vi "Configure Trigger (Runt).vi"(0 "VISA resource name":refnum<visa-resource-name>, 1 "Polarity (0:Positive)":u16(ring) items=["Positive", "Negative", "Either"], 2 "Upper Level (1.2V)":dbl=1.2, 3 "Lower Level (0.8V)":dbl=0.8, 5 "Source (0:Channel1)":u16(ring) items=["Channel1", "Channel2", "Channel3", "Channel4", "Digital Channel0", "Digital Channel1", "Digital Channel2", "Digital Channel3", "Digital Channel4", "Digital Channel5", "Digital Channel6", "Digital Channel7", "Digital Channel8", "Digital Channel9", "Digital Channel10", "Digital Channel11", "Digital Channel12", "Digital Channel13", "Digital Channel14", "Digital Channel15"], 7 "Trigger Condition (1: Wider than)":u16(ring)=1 items=["Occurs", "Wider Than"], 9 "Runt Width (500E-12s)":dbl=5e-10, 11 "error in (no error)":errorcluster, 12 "Trigger if Runt (0:Occurs)":u16(ring) items=["Occurs", "Logic", "Bus"], 13 "Trigger Event (0:A Event)":u16(ring) items=["A Event", "B Event"]) -> (4 "VISA resource name out":refnum<visa-resource-name>, 6 "Trigger Event Out":u16(ring) items=["A Event", "B Event"], 15 "error out":errorcluster)   [LabVIEW 2012, in "Tektronix 7000 Series.lvlib"]
doc: "Configures Runt trigger settings for an oscilloscope.A runt occurs when the oscilloscope detects a positive or negative going pulse that crosses one voltage threshold but fails to cross a second threshold before re-crossing the first. \n\nTDS5000,TDS5000B,TDS6000,CSA7000 and TDS7000 series oscilloscopes don't support B Runt Trigger."
uses:
  Tektronix 7000 Series.lvlib
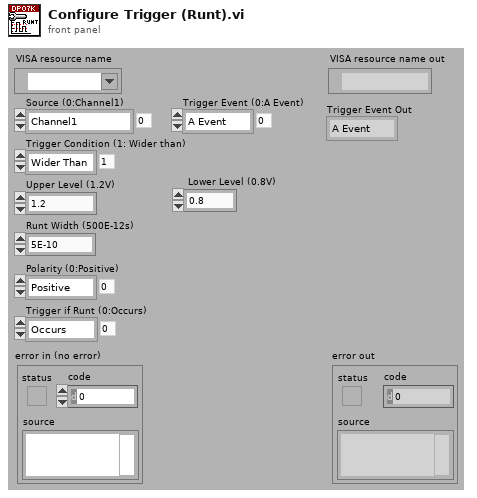
[diagram p1: front panel]
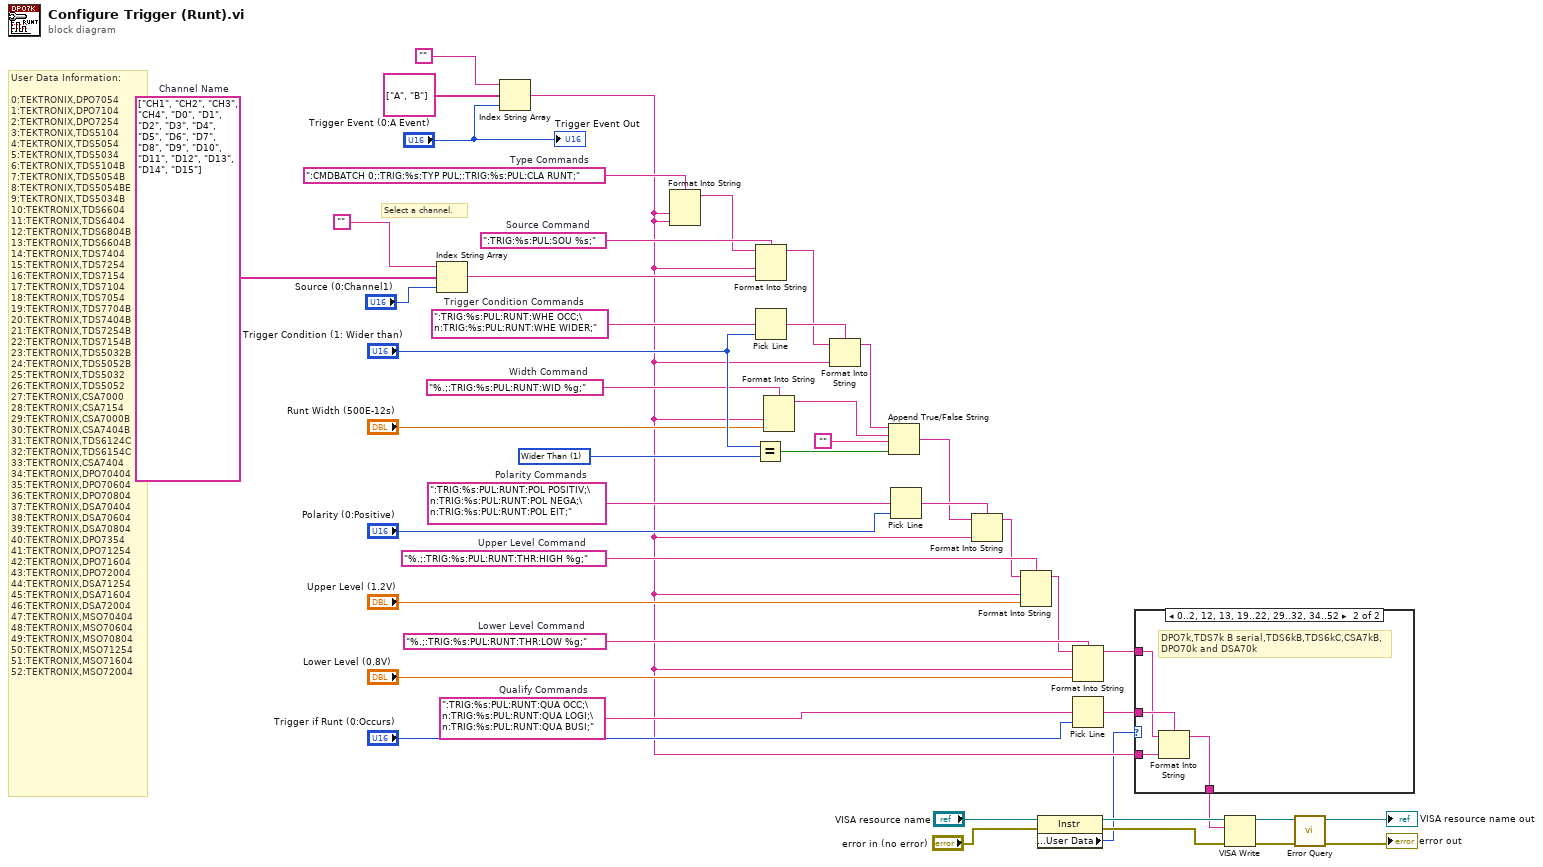
[diagram p0: block diagram]
diagram:
  w1 = string[] ["CH1", "CH2", "CH3", "CH4", "D0", "D1", "D2", "D3", "D4", "D5", "D6", "D7", "D8", "D9", "D10", "D11", "D12", "D13", "D14", "D15"]  # Channel Name
  w27 = "%.;:TRIG:%s:PUL:RUNT:WID %g;"  # Width Command
  w28 = u16 1 items=["Occurs", "Wider Than"] ("Trigger Condition (1: Wider than)")
  w30 = ":TRIG:%s:PUL:RUNT:QUA OCC;\n:TRIG:%s:PUL:RUNT:QUA LOGI;\n:TRIG:%s:PUL:RUNT:QUA BUSI;"  # Qualify Commands
  w31 = ":TRIG:%s:PUL:RUNT:POL POSITIV;\n:TRIG:%s:PUL:RUNT:POL NEGA;\n:TRIG:%s:PUL:RUNT:POL EIT;"  # Polarity Commands
  w33 = ":TRIG:%s:PUL:RUNT:WHE OCC;\n:TRIG:%s:PUL:RUNT:WHE WIDER;"  # Trigger Condition Commands
  w32 = "%.;:TRIG:%s:PUL:RUNT:THR:LOW %g;"  # Lower Level Command
  w34 = "%.;:TRIG:%s:PUL:RUNT:THR:HIGH %g;"  # Upper Level Command
  w35 = ":TRIG:%s:PUL:SOU %s;"  # Source Command
  w23 = ":CMDBATCH 0;:TRIG:%s:TYP PUL;:TRIG:%s:PUL:CLA RUNT;"  # Type Commands
  # "User Data Information:\n\n0:TEKTRONIX,DPO7054\n1:TEKTRONIX,DPO7104\n2:TEKTRONIX,DPO7254\n3:TEKTRONIX,TDS5104\n4:TEKTRONIX,TDS5054\n5:TEKTRONIX,TDS5034\n6:TEKTRONIX,TDS5104B\n7:TEKTRONIX,TDS5054B\n8:TEKTRONIX,TDS5054BE\n9:TEKTRONIX,TDS5034B\n10:TEKTRONIX,TDS6604\n11:TEKTRONIX,TDS6404\n12:TEKTRONIX,TDS6804B\n13:TEKTRONIX,TDS6604B\n14:TEKTRONIX,TDS7404\n15:TEKTRONIX,TDS7254\n16:TEKTRONIX,TDS7154\n17:TEKTRONIX,TDS7104\n18:TEKTRONIX,TDS7054\n19:TEKTRONIX,TDS7704B\n20:TEKTRONIX,TDS7404B\n21:TEKTRONIX,TDS7254B\n22:TEKTRONIX,TDS7154B\n23:TEKTRONIX,TDS5032B\n24:TEKTRONIX,TDS5052B\n25:TEKTRONIX,TDS5032\n26:TEKTRONIX,TDS5052\n27:TEKTRONIX,CSA7000\n28:TEKTRONIX,CSA7154\n29:TEKTRONIX,CSA7000B\n30:TEKTRONIX,CSA7404B\n31:TEKTRONIX,TDS6124C\n32:TEKTRONIX,TDS6154C\n33:TEKTRONIX,CSA7404\n34:TEKTRONIX,DPO70404\n35:TEKTRONIX,DPO70604\n36:TEKTRONIX,DPO70804\n37:TEKTRONIX,DSA70404\n38:TEKTRONIX,DSA70604\n39:TEKTRONIX,DSA70804\n40:TEKTRONIX,DPO7354\n41:TEKTRONIX,DPO71254\n42:TEKTRONIX,DPO71604\n43:TEKTRONIX,DPO72004\n44:TEKTRONIX,DSA71254\n45:TEKTRONIX,DSA71604\n46:TEKTRONIX,DSA72004\n47:TEKTRONIX,MSO70404\n48:TEKTRONIX,MSO70604\n49:TEKTRONIX,MSO70804\n50:TEKTRONIX,MSO71254\n51:TEKTRONIX,MSO71604\n52:TEKTRONIX,MSO72004"
  # "Select a channel."
  n1 = Index String Array(1:"Source (0:Channel1)", 2:w1, 3:"" ("Empty String Constant")) -> (0:w22:string)
  n2 = Index String Array(1:"Trigger Event (0:A Event)", 2:string[] ["A", "B"], 3:"" ("Empty String Constant")) -> (0:w6:string)
  n3 = Format Into String(format string=w23, w6, w6) -> (resulting string=w21:string)  [unwired: 2 in, 1 out]
  n4 = Equal?(x="Trigger Condition (1: Wider than)", y=w28) -> (x = y?=w26:bool)
  n5 = Format Into String(format string=w35, initial string=w21, w6, w22) -> (resulting string=w19:string)  [unwired: 1 in, 1 out]
  n6 = Pick Line(multi-line string=w33, line index="Trigger Condition (1: Wider than)") -> (output string=w20:string)  [unwired: 1 in]
  n7 = Format Into String(format string=w27, w6, "Runt Width (500E-12s)") -> (resulting string=w25:string)  [unwired: 2 in, 1 out]
  n8 = Format Into String(format string=w20, initial string=w19, w6) -> (resulting string=w17:string)  [unwired: 1 in, 1 out]
  n9 = Append True/False String(1:w26, 2:"" ("Empty String Constant"), 3:w25, 4:w17) -> (0:w15:string)
  n10 = Pick Line(multi-line string=w31, line index="Polarity (0:Positive)") -> (output string=w16:string)  [unwired: 1 in]
  n11 = Format Into String(format string=w16, initial string=w15, w6) -> (resulting string=w7:string)  [unwired: 1 in, 1 out]
  n12 = Format Into String(format string=w34, initial string=w7, w6, "Upper Level (1.2V)") -> (resulting string=w29:string)  [unwired: 1 in, 1 out]
  n13 = property class="Instr"(reference="VISA resource name", error in="error in (no error)") -> (reference out=w10:refnum<visa-resource-name>, error out=w9:errorcluster, "General Settings:User Data"=w5:u32)
  n14 = Format Into String(format string=w32, initial string=w29, w6, "Lower Level (0.8V)") -> (resulting string=w4:string)  [unwired: 1 in, 1 out]
  n15 = Pick Line(multi-line string=w30, line index="Trigger if Runt (0:Occurs)") -> (output string=w13:string)  [unwired: 1 in]
  n16 = case shown="0..2, 12, 13, 19..22, 29..32, 34..52" w5 {
    tunnel: w13 -> [_ w51]
    tunnel: w6 -> [_ w50]
    tunnel: w4 -> [w47 w49]
    tunnel: [w47 w48] -> w3
    frame Default {
    }
    frame 0..2, 12, 13, 19..22, 29..32, 34..52 {
      # "DPO7k,TDS7k B serial,TDS6kB,TDS6kC,CSA7kB,\nDPO70k and DSA70k"
      n17 = Format Into String(format string=w51, initial string=w49, w50) -> (resulting string=w48:string)  [unwired: 1 in, 1 out]
    }
  }
  n18 = VISA Write(VISA resource name=w10, write buffer=w3, error in (no error)=w9) -> (VISA resource name out=w40:refnum<visa-resource-name>, error out=w41:errorcluster)  [unwired: 1 out]
  n19 = call "Error Query.vi"("error in (no error)"=w41, "VISA resource name"=w40) -> ("error out"=→"error out":errorcluster, "VISA resource name out"=→"VISA resource name out":refnum<visa-resource-name>)  [unwired: 6 in, 2 out]
  "Trigger Event Out" <- "Trigger Event (0:A Event)"
